vi "myRIO_BRig_Host_v0,12.vi"() -> ()   [LabVIEW 2014]
panel:
  out "output_I_data 2":bool
  out "output_I_data":bool
  out "BlockL_T2R_cur":u16 caption="Trials2Reward"
  out "BlockL_BTPR_cur":u16 caption="BadTrialsPostReward"
  out "BlockL_T2R_avg":dbl caption="Trials2Reward" format="%#_3g"
  out "BlockL_BTPR_avg":dbl caption="BadTrialsPostReward" format="%#_3g"
  out "BlockR_T2R_cur":u16 caption="Trials2Reward"
  out "BlockR_BTPR_cur":u16 caption="BadTrialsPostReward"
  out "BlockR_T2R_avg":dbl caption="Trials2Reward" format="%#_3g"
  out "BlockR_BTPR_avg":dbl caption="BadTrialsPostReward" format="%#_3g"
  out "RunTime_minutes":u16
  out "RunTime_seconds":u16
  out "error out 2":errorcluster caption="error out"
  in  "dataIn_maxTrialsDisplayed":u16 caption="Number of Trials Displayed\n( 0 = all trials )"
  in  "colorIn_timeout":u32(colorbox)=7468543 caption="Choice Timeout"
  in  "colorIn_wrong/cue":u32(colorbox)=16728618 caption="Wrong Choice or\nLicked During Cue"
  in  "colorIn_reward":u32(colorbox)=5898088 caption="Reward"
  in  "colorIn_unknown":u32(colorbox)=16449331 caption="Unknown Trial Status"
  in  "LoadPrevSettings":bool
  out "dataOut_plot":cluster{i32[], i32[]}[](graph)
  out "iBlock":u16
  out "iTrial":u16
  in  "stop":bool
  # "Exp Stats"
  # "Current Block Stats"
  # "Trials 2 Reward\n\nBad Trials\nPost Reward"
  # "Left Spout    Right Spout"
  # "Run Time\n\n   minutes    seconds"
  # "Average Block Stats"
  # "Trials 2 Reward\n\nBad Trials\nPost Reward"
  # "Left Spout    Right Spout"
  # "If you get ERROR 5 related to opening a file, press CONTINUE"
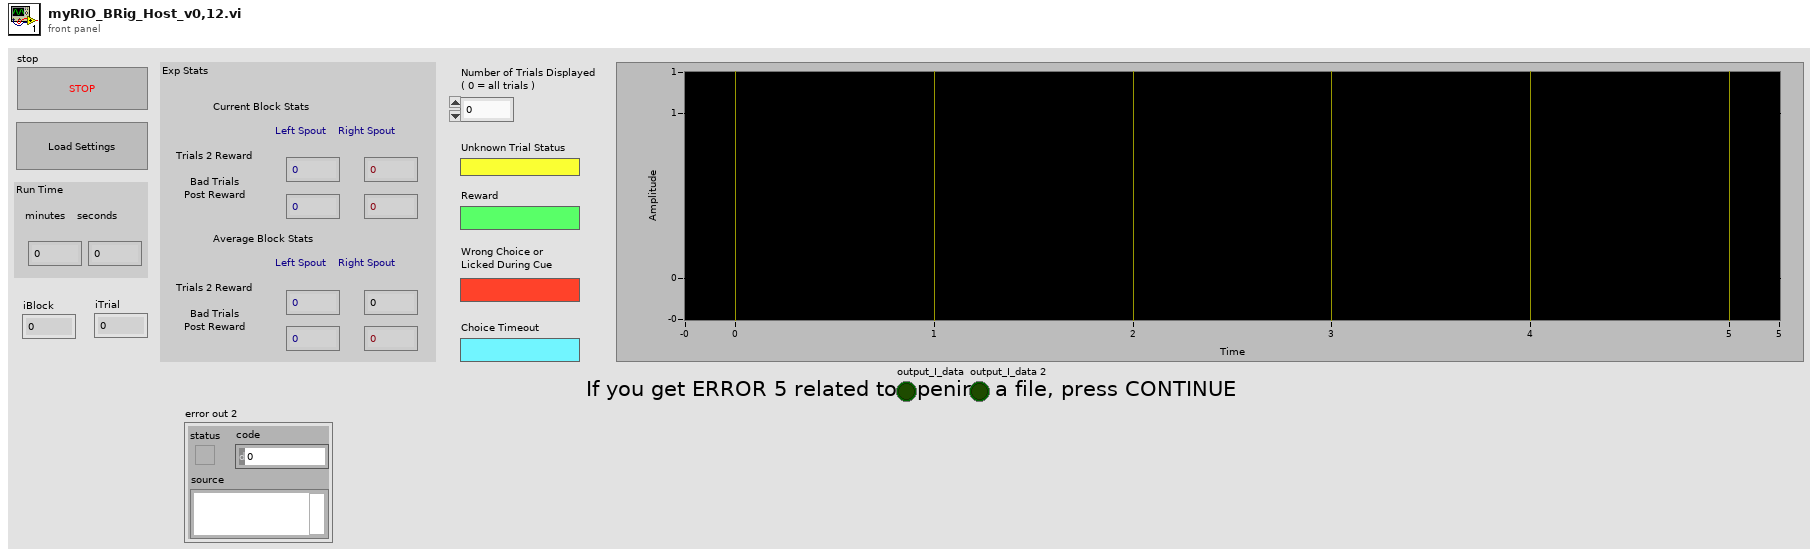
[diagram p1: front panel]
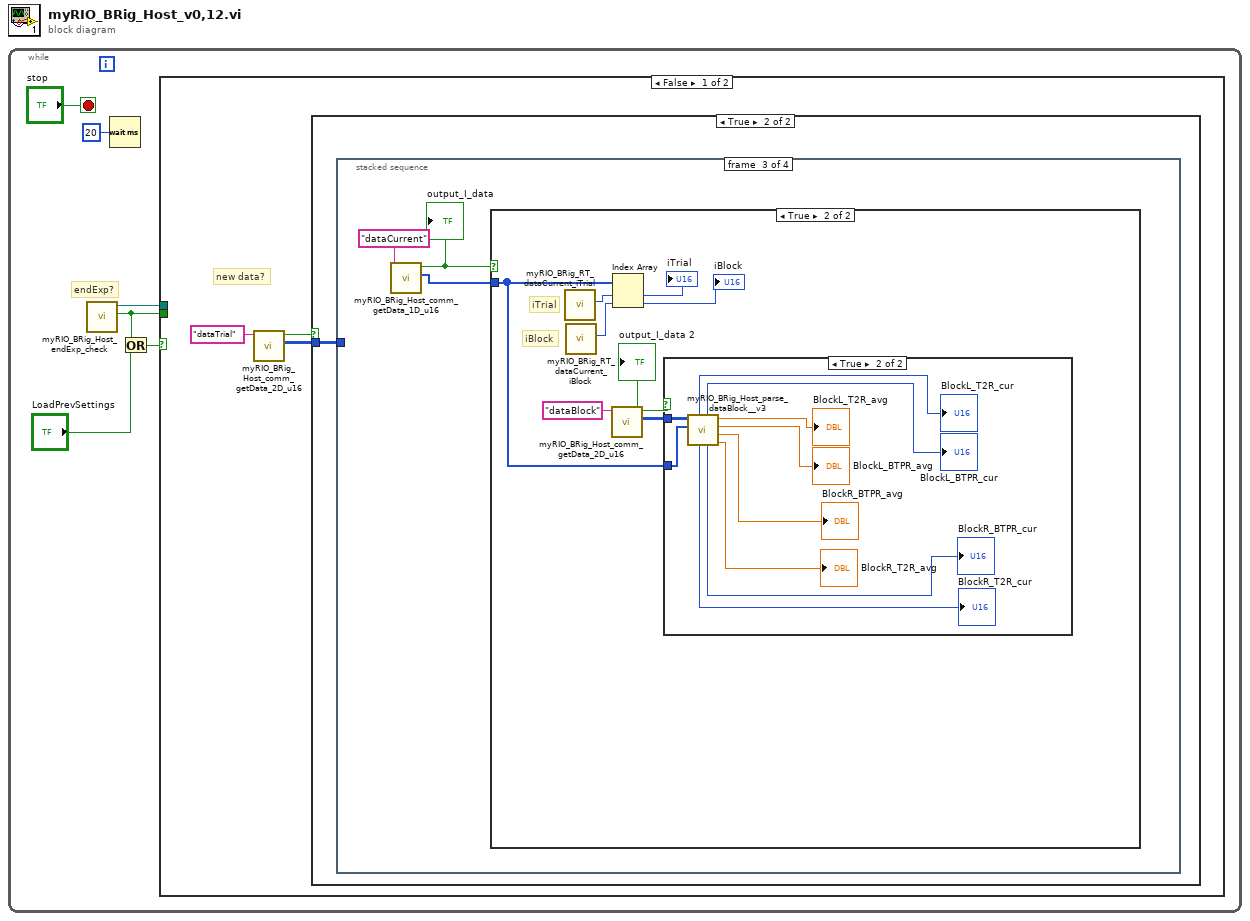
[diagram p0: block diagram]
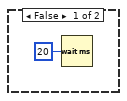
[diagram p2: hidden frame]
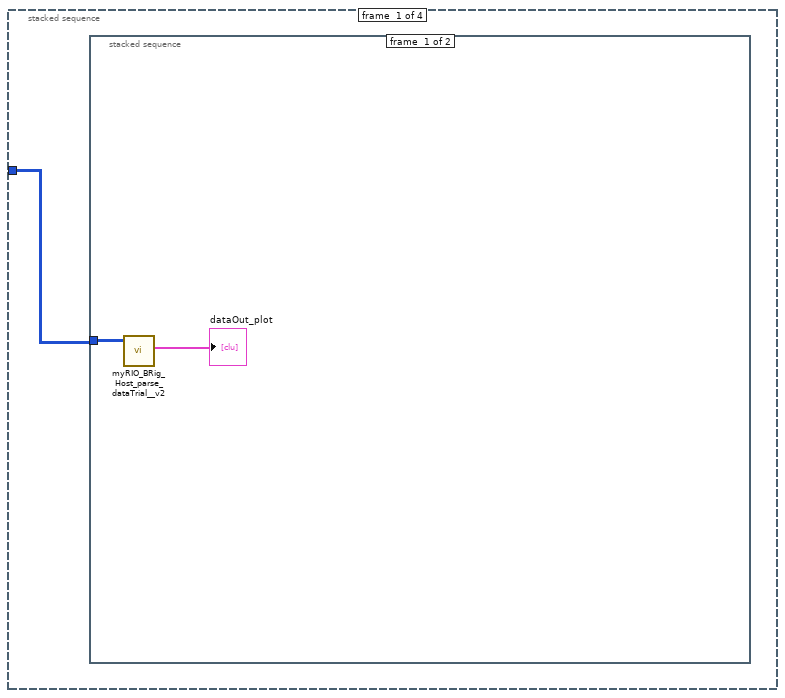
[diagram p3: hidden frame]
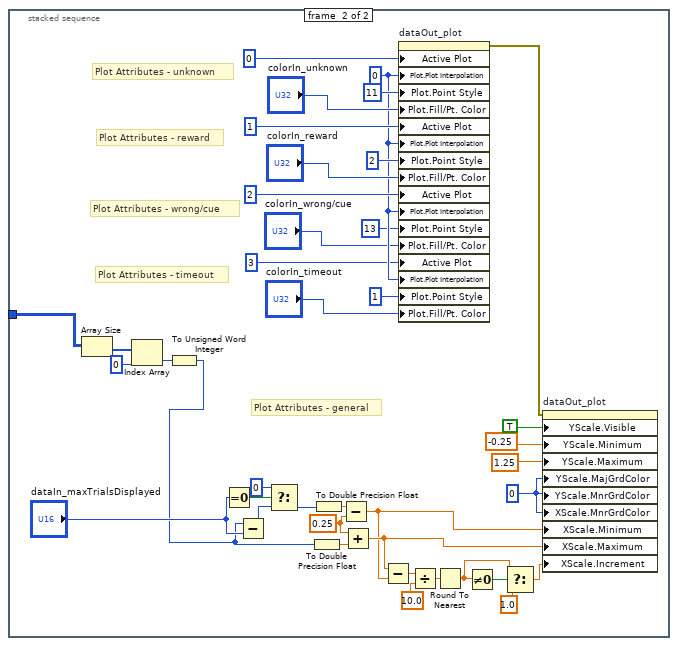
[diagram p4: hidden frame]
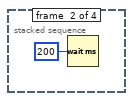
[diagram p5: hidden frame]
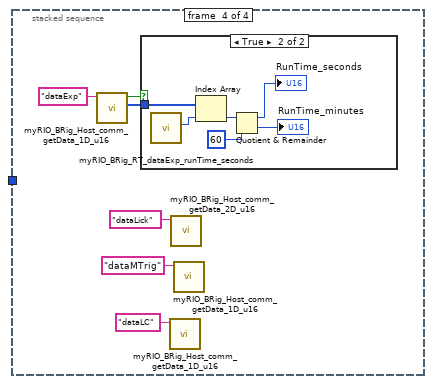
[diagram p8: hidden frame]
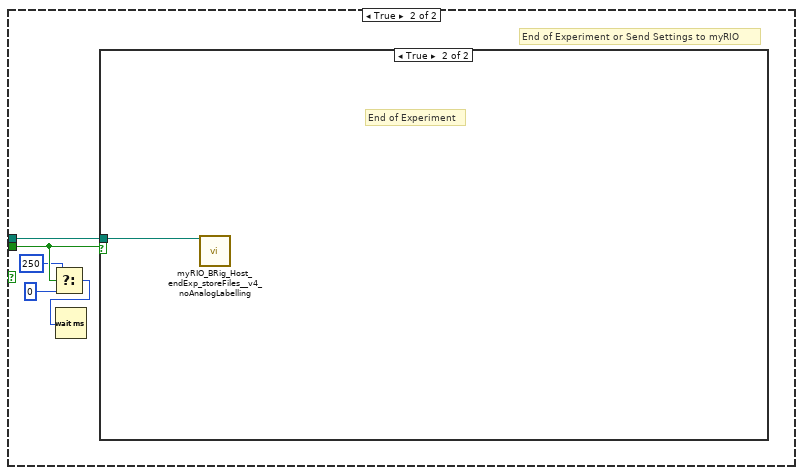
[diagram p10: hidden frame]
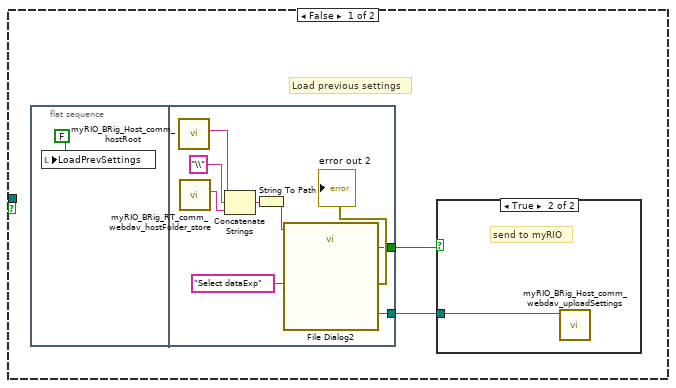
[diagram p11: hidden frame]
diagram:
  n1 = while {
    stop <- "stop" stop-if-true
    # "endExp?"
    n2 = call "myRIO_BRig_Host_endExp_check.vi"() -> ("output_IendExp"=w3:bool, "output_filePath_expExp"=w2:path)  [unwired: 10 in]
    n3 = Wait (ms)(milliseconds to wait=u32 20) -> ()  [unwired: 1 out]
    n4 = Or(x=w3, y="LoadPrevSettings") -> (x .or. y?=w4:bool)
    n5 = case shown="False" w4 {
      tunnel: w3 -> [_ w92]
      tunnel: w2 -> [_ w93]
      frame False {
        # "new data?"
        n6 = call "myRIO_BRig_Host_comm_getData_2D_u16.vi"("input_fileName"="dataTrial") -> ("output_data_2D"=w7:u16[][], "output_I_data"=w8:bool)  [unwired: 9 in]
        n7 = case shown="True" w8 {
          tunnel: w7 -> [_ w11]
          frame False {
            n8 = Wait (ms)(milliseconds to wait=u32 20) -> ()  [unwired: 1 out]
          }
          frame True {
            n9 = stacked-sequence {
              tunnel: w11 -> [w12 _ _ _]
              frame #0 {
                n10 = stacked-sequence {
                  tunnel: w12 -> [w13 w19]
                  frame #0 {
                    n11 = call "myRIO_BRig_Host_parse_dataTrial__v2.vi"("arrayIn_dataTrial"=w13) -> ("appended array"=→"dataOut_plot":cluster{i32[], i32[]}[])  [unwired: 10 in]
                  }
                  frame #1 {
                    w34 = 0.25 ("y")
                    w38 = u32 0 ("Y Scale.Grid Colors:Major Color")
                    w47 = u8 0 ("Plot.Plot Interpolation")
                    # "Plot Attributes - general"
                    # "Plot Attributes - timeout"
                    # "Plot Attributes - wrong/cue"
                    # "Plot Attributes - reward"
                    # "Plot Attributes - unknown"
                    n12 = Array Size(array=w19) -> (size(s)=w21:i32[])
                    n13 = Index Array(array=w21, index=0) -> (element=w17:i32)
                    n14 = To Unsigned Word Integer(number=w17) -> (unsigned 16bit integer=w16:u16)
                    n15 = Equal To 0?(x="dataIn_maxTrialsDisplayed") -> (x = 0?=w37:bool)
                    n16 = Subtract(x=w16, y="dataIn_maxTrialsDisplayed") -> (x-y=w36:u16)
                    n17 = Select(t=u16 0, s=w37, f=w36) -> (s? t:f=w31:u16)
                    n18 = To Double Precision Float(number=w16) -> (double precision float=w33:dbl)
                    n19 = To Double Precision Float(number=w31) -> (double precision float=w32:dbl)
                    n20 = Subtract(x=w32, y=w34) -> (x-y=w23:dbl)
                    n21 = Add(x=w34, y=w33) -> (x+y=w24:dbl)
                    n22 = Subtract(x=w24, y=w23) -> (x-y=w30:dbl)
                    n23 = property on="dataOut_plot" class="XYGraph (strict)"("Active Plot"=u32 0, "Plot.Plot Interpolation"=w47, "Plot.Point Style"=u8 11, "Plot.Fill/Pt. Color"="colorIn_unknown", "Active Plot"=u32 1, "Plot.Plot Interpolation"=w47, "Plot.Point Style"=u8 2, "Plot.Fill/Pt. Color"="colorIn_reward", "Active Plot"=u32 2, "Plot.Plot Interpolation"=w47, "Plot.Point Style"=u8 13, "Plot.Fill/Pt. Color"="colorIn_wrong/cue", "Active Plot"=u32 3, "Plot.Plot Interpolation"=w47, "Plot.Point Style"=u8 1, "Plot.Fill/Pt. Color"="colorIn_timeout") -> (error out=w22:errorcluster)  [unwired: 2 in, 1 out]
                    n24 = Divide(x=w30, y=10.0) -> (x/y=w28:dbl)
                    n25 = Round To Nearest(number=w28) -> (nearest integer value=w26:dbl)
                    n26 = Not Equal To 0?(x=w26) -> (x != 0?=w27:bool)
                    n27 = Select(t=w26, s=w27, f=1.0) -> (s? t:f=w25:dbl)
                    n28 = property on="dataOut_plot" class="XYGraph (strict)"(error in=w22, "YScale.Visible"=TRUE ("Y Scale.Visible"), "YScale.Minimum"=-0.25 ("Y Scale.Range:Minimum"), "YScale.Maximum"=1.25 ("Y Scale.Range:Maximum"), "YScale.MajGrdColor"=w38, "YScale.MnrGrdColor"=w38, "XScale.MnrGrdColor"=w38, "XScale.Minimum"=w23, "XScale.Maximum"=w24, "XScale.Increment"=w25) -> ()  [unwired: 1 in, 2 out]
                  }
                }
              }
              frame #1 {
                n29 = Wait (ms)(milliseconds to wait=u32 200) -> ()  [unwired: 1 out]
              }
              frame #2 {
                n30 = call "myRIO_BRig_Host_comm_getData_1D_u16.vi"("input_fileName"="dataCurrent") -> ("output_data_1D"=w56:u16[], "output_I_data"=w57:bool)  [unwired: 9 in]
                "output_I_data" <- w57
                n31 = case shown="True" w57 {
                  tunnel: w56 -> [_ w59]
                  frame False {
                  }
                  frame True {
                    # "iBlock"
                    # "iTrial"
                    n32 = call "myRIO_BRig_RT_dataCurrent_iTrial.vi"() -> ("output_iTrial"=w66:i32)  [unwired: 11 in]
                    n33 = call "myRIO_BRig_RT_dataCurrent_iBlock.vi"() -> ("output_iBlock"=w65:i32)  [unwired: 11 in]
                    n34 = call "myRIO_BRig_Host_comm_getData_2D_u16.vi"("input_fileName"="dataBlock") -> ("output_data_2D"=w60:u16[][], "output_I_data"=w61:bool)  [unwired: 9 in]
                    "output_I_data 2" <- w61
                    n35 = Index Array(array=w59, index #1=w66, index #2=w65) -> (element #1=→"iTrial":u16, element #2=→"iBlock":u16)
                    n36 = case shown="True" w61 {
                      tunnel: w60 -> [_ w68]
                      tunnel: w59 -> [_ w67]
                      frame False {
                      }
                      frame True {
                        n37 = call "myRIO_BRig_Host_parse_dataBlock__v3.vi"("input_dataCurrent"=w67, "input_dataBlock"=w68) -> ("BlockR_T2R_avg"=→"BlockR_T2R_avg":dbl, "BlockR_BTPR_avg"=→"BlockR_BTPR_avg":dbl, "BlockL_BTPR_avg"=→"BlockL_BTPR_avg":dbl, "BlockL_T2R_avg"=→"BlockL_T2R_avg":dbl, "BlockR_BTPR_cur"=→"BlockR_BTPR_cur":u16, "BlockL_BTPR_cur"=→"BlockL_BTPR_cur":u16, "BlockR_T2R_cur"=→"BlockR_T2R_cur":u16, "BlockL_T2R_cur"=→"BlockL_T2R_cur":u16)  [unwired: 2 in]
                      }
                    }
                  }
                }
              }
              frame #3 {
                n38 = call "myRIO_BRig_Host_comm_getData_1D_u16.vi"("input_fileName"="dataExp") -> ("output_data_1D"=w80:u16[], "output_I_data"=w81:bool)  [unwired: 9 in]
                n39 = case shown="True" w81 {
                  tunnel: w80 -> [_ w88]
                  frame False {
                  }
                  frame True {
                    n40 = call "myRIO_BRig_RT_dataExp_runTime_seconds.vi"() -> ("output_RunTime_minutes"=w87:i32)  [unwired: 11 in]
                    n41 = Index Array(array=w88, index=w87) -> (element=w86:u16)
                    n42 = Quotient & Remainder(x=w86, y=u16 60) -> (x-y*floor(x/y)=→"RunTime_seconds":u16, floor(x/y)=→"RunTime_minutes":u16)
                  }
                }
                n43 = call "myRIO_BRig_Host_comm_getData_1D_u16.vi"("input_fileName"="dataLC") -> ()  [unwired: 9 in, 2 out]
                n44 = call "myRIO_BRig_Host_comm_getData_2D_u16.vi"("input_fileName"="dataLick") -> ()  [unwired: 9 in, 2 out]
                n45 = call "myRIO_BRig_Host_comm_getData_1D_u16.vi"("input_fileName"="dataMTrig") -> ()  [unwired: 9 in, 2 out]
              }
            }
          }
        }
      }
      frame True {
        # "End of Experiment or Send Settings to myRIO"
        n46 = Select(t=u32 250 ("milliseconds to wait"), s=w92, f=u32 0 ("milliseconds to wait")) -> (s? t:f=w90:u32)
        n47 = Wait (ms)(milliseconds to wait=w90) -> ()  [unwired: 1 out]
        n48 = case shown="True" w92 {
          tunnel: w93 -> [_ w107]
          frame False {
            # "Load previous settings"
            n49 = flat-sequence {
              tunnel: [w99] -> w94
              tunnel: [w98] -> w95
              frame #0 {
                n50 = local write "LoadPrevSettings"(FALSE ("LoadPrevSettings")) -> ()
              }
              frame #1 {
                n51 = call "myRIO_BRig_Host_comm_hostRoot.vi"() -> ("output_hostRoot"=w101:string)  [unwired: 11 in]
                n52 = call "myRIO_BRig_RT_comm_webdav_hostFolder_store.vi"() -> ("output_HostFolder"=w103:string)  [unwired: 11 in]
                n53 = Concatenate Strings(w101, "\\" ("string"), w103) -> (w105:string)
                n54 = String To Path(string=w105) -> (path=w104:path)
                n55 = call "File Dialog2"("start path"=w104, "prompt"="Select dataExp") -> ("selected path"=w99:path, "exists"=w98:bool, "error out"=→"error out 2":errorcluster)  [unwired: 10 in, 1 out]
              }
            }
            n56 = case shown="True" w95 {
              tunnel: w94 -> [_ w96]
              frame False {
                # "invalid file\nor\ncancelled"
              }
              frame True {
                # "send to myRIO"
                n57 = call "myRIO_BRig_Host_comm_webdav_uploadSettings.vi"("input_filePath"=w96) -> ()  [unwired: 11 in]
              }
            }
          }
          frame True {
            # "End of Experiment"
            n58 = call "myRIO_BRig_Host_endExp_storeFiles__v4_noAnalogLabelling.vi"("input_filePath"=w107) -> ()  [unwired: 15 in]
          }
        }
      }
    }
  }
